vi "MoveXYRelative_Striptest.vi"(8 "error in (no error)":errorcluster, 9 "Y_Offset":dbl, 10 "X_Offset":dbl, 11 "ProbeStationControl in":refnum<class "ProbeStationControl.lvclass">) -> (0 "error out":errorcluster, 3 "ProbeStationControl out 2":refnum<class "ProbeStationControl.lvclass">)   [LabVIEW 2019]
uses:
  itk-strip-sensor-qc/LabVIEW 2019/InstrControl/ProbeStationControl/ProbeStationControl.lvclass
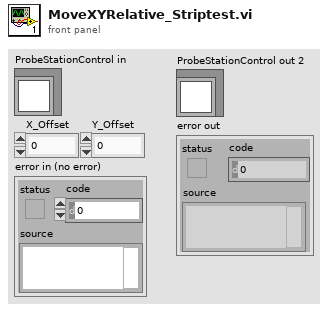
[diagram p1: front panel]
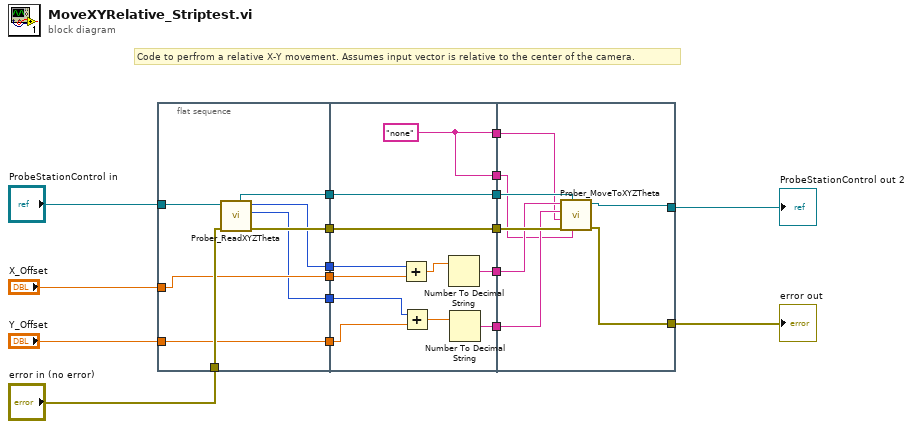
[diagram p0: block diagram]
diagram:
  # "Code to perfrom a relative X-Y movement. Assumes input vector is relative to the center of the camera."
  n1 = flat-sequence {
    tunnel: "ProbeStationControl in" -> [w26]
    tunnel: [w25] -> w16
    tunnel: "error in (no error)" -> [w24]
    tunnel: [w23] -> w12
    tunnel: "X_Offset" -> [w22]
    tunnel: [w22] -> w9
    tunnel: [w21] -> w8
    tunnel: "Y_Offset" -> [w21]
    tunnel: [w20] -> w6
    tunnel: [w19] -> w5
    tunnel: [w37] -> w17
    tunnel: w16 -> [w37]
    tunnel: [w36] -> w13
    tunnel: w12 -> [w36]
    tunnel: w9 -> [w35]
    tunnel: w8 -> [w34]
    tunnel: w6 -> [w33]
    tunnel: w5 -> [w32]
    tunnel: [w29] -> w4
    tunnel: [w28] -> w3
    tunnel: [w27] -> w2
    tunnel: [w27] -> w1
    tunnel: w17 -> [w45]
    tunnel: [w44] -> w15
    tunnel: w13 -> [w43]
    tunnel: [w42] -> w11
    tunnel: w4 -> [w41]
    tunnel: w3 -> [w40]
    tunnel: w2 -> [w39]
    tunnel: w1 -> [w38]
    frame #0 {
      n2 = call-dynamic "Prober_ReadXYZTheta.vi"("error in (no error)"=w24, "ProbeStationControl in"=w26) -> ("error out"=w23:errorcluster, "Y location [µm]"=w19:i32, "X location [µm]"=w20:i32, "ProbeStationControl out"=w25:refnum<class "ProbeStationControl.lvclass">)  [unwired: 4 in, 2 out]
    }
    frame #1 {
      w27 = "none"
      n3 = Add(x=w33, y=w35) -> (x+y=w31:dbl)
      n4 = Add(x=w32, y=w34) -> (x+y=w30:dbl)
      n5 = Number To Decimal String(number=w31) -> (decimal integer string=w29:string)  [unwired: 1 in]
      n6 = Number To Decimal String(number=w30) -> (decimal integer string=w28:string)  [unwired: 1 in]
    }
    frame #2 {
      n7 = call-dynamic "Prober_MoveToXYZTheta.vi"("Theta location [mdeg]"=w38, "ProbeStationControl in"=w45, "error in (no error)"=w43, "Z location [µm]"=w39, "Y location [µm]"=w40, "X location [µm]"=w41) -> ("error out"=w42:errorcluster, "ProbeStationControl out"=w44:refnum<class "ProbeStationControl.lvclass">)  [unwired: 3 in, 1 out]
    }
  }
  "ProbeStationControl out 2" <- w15
  "error out" <- w11
